vi "Register DI IRQ.vi"(4 "Callback VI Reference":T1, 6 "Edge Count":u32=1, 8 "error in (no error)":errorcluster, 9 "Digital Interrupt Type":T2, 10 "Channel Name":tag, 11 "IRQ Number":u8) -> (0 "error out":errorcluster)   [LabVIEW 2021, in "IO IRQ.lvlib"]
uses:
  <vilib>/myRIO/Instrument Drivers/IRQ/IO IRQ/IO IRQ.lvlib
  <vilib>/myRIO/Common/Instrument Driver Framework/myRIO v1.0/IRQ/typedefs/Callback VI Ref.ctl
  <vilib>/myRIO/Common/Instrument Driver Framework/myRIO v1.0/IRQ/typedefs/DI IRQ Type.ctl
  <vilib>/myRIO/Instrument Drivers/IRQ/IO IRQ/vis/myRIO Register DI IRQ.xnode
  <vilib>/userdefined/High Color/nirio_resource_hc.ctl
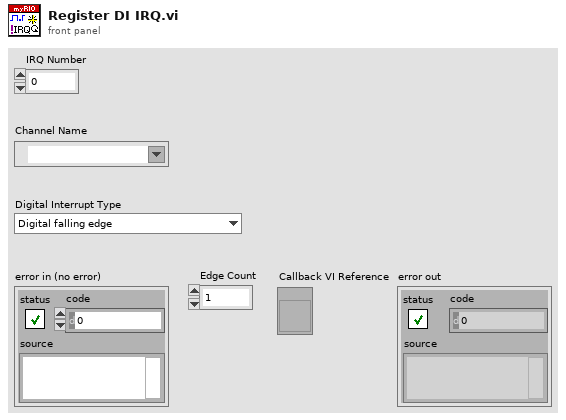
[diagram p1: front panel]
types:
  T1 = typedef "Callback VI Ref.ctl" = refnum<vi>
  T2 = typedef "DI IRQ Type.ctl" = enum16{"Digital falling edge", "Digital rising edge", "Digital edge"}
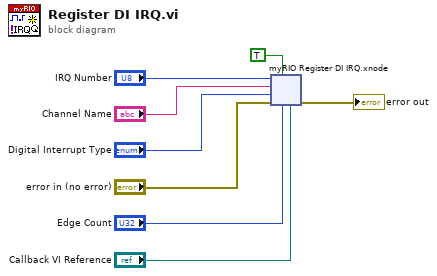
[diagram p0: block diagram]
diagram:
  n1 = xnode "myRIO Register DI IRQ.xnode"("error in (no error)"="error in (no error)", "Channel Name"="Channel Name", "Callback VI Reference"="Callback VI Reference", "Allow Overwrite Operation? (F)"=TRUE ("Allow Overwrite? (F)"), "Edge Count"="Edge Count", "IRQ Number"="IRQ Number", "Digital Interrupt Type"="Digital Interrupt Type") -> ("error out"=→"error out":errorcluster)
